vi "Init_Test.vi"(8 "error in (no error)":errorcluster caption="entrée d'erreur (pas d'erreur)", 11 "Get_Voltage en entrée":refnum<class "Close_ShieldingBox.lvclass">) -> (0 "error out":errorcluster caption="sortie d'erreur", 3 "Get_Voltage en sortie":refnum<class "Close_ShieldingBox.lvclass">)   [LabVIEW 2020, in "Library Test.lvlib" / "Close_ShieldingBox.lvclass"]
uses:
  Close_ShieldingBox.lvclass
  C:/Users/ngarcin/OneDrive - Altyor/Standard TB/Class/Test/Test (Default)/Test (Default).lvclass
  Commun VI/TypeDef/Commande Test/Commande Value Type.ctl
  Commun VI/TypeDef/Commande Test/Commande Type Test.ctl
  Test/Test_Wtih_Instr/Test_With_Inst.lvclass
  Close_ShieldingBox.lvclass/Close_ShieldingBox.ctl
  Commun VI/Library Commun.lvlib
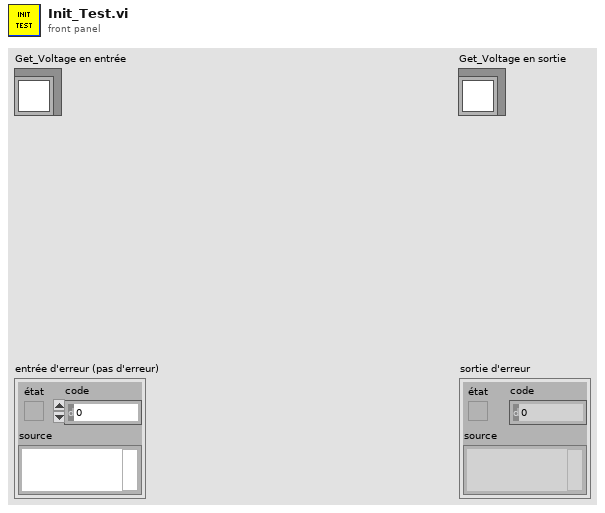
[diagram p1: front panel]
types:
  T1 = typedef "Library Commun.lvlib/Commande Type Test.ctl" = enum16{"Function", "Test", "Calculation"}
  T2 = typedef "Library Commun.lvlib/Commande Value Type.ctl" = enum16{"None", "String", "Number", "Timestamp", "Boolean", "Array"}
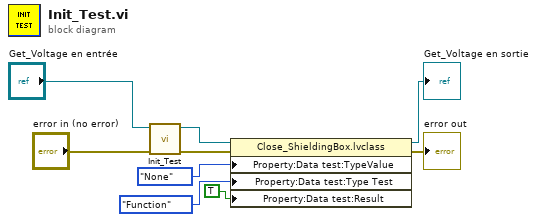
[diagram p0: block diagram]
diagram:
  n1 = call-parent "Init_Test.vi"("error in (no error)"="error in (no error)", "Test_With_Inst en entrée"="Get_Voltage en entrée") -> ("error out"=w6:errorcluster, "Test_With_Inst en sortie"=w7:refnum<class "Close_ShieldingBox.lvclass">)  [unwired: 8 in]
  n2 = property class="Close_ShieldingBox.lvclass"(reference=w7, error in=w6, "Property:Data test:TypeValue"=Commande_Value_Type."None" ("TypeValue"), "Property:Data test:Type Test"=Commande_Type_Test."Function" ("Type Test"), "Property:Data test:Result"=TRUE ("Result")) -> (reference out=→"Get_Voltage en sortie":refnum<class "Close_ShieldingBox.lvclass">, error out=→"error out":errorcluster)
